vi "OCT Configuration Typedef.vi"() -> ()   [LabVIEW 2014]
uses:
  Classes/D to A/External Clock.lvclass
  Classes/Galvo/Galvo.lvclass
  Classes/Laser/Laser.lvclass
  Classes/DAQ/DAQ Class.lvclass
panel:
  in  "Cluster":T1
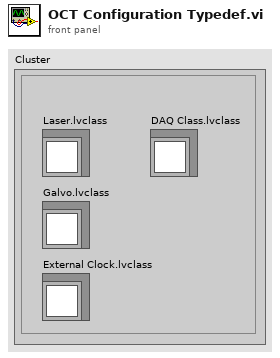
[diagram p1: front panel]
types:
  T1 = cluster{"External Clock.lvclass":refnum<class "External Clock.lvclass">, "Galvo.lvclass":refnum<class "Galvo.lvclass">, "Laser.lvclass":refnum<class "Laser.lvclass">, "DAQ Class.lvclass":refnum<class "DAQ Class.lvclass">}
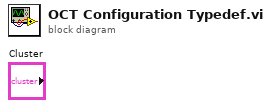
[diagram p0: block diagram]
diagram:
